vi "Disconnect.vi"(8 "error in (no error)":errorcluster, 11 "TCP Comm":T1) -> (0 "error out":errorcluster)   [LabVIEW 2020, in "TCP Comms.lvlib"]
uses:
  TCP Comms.lvlib
  TCP Comm.ctl
  Ref Data.ctl
  State.ctl
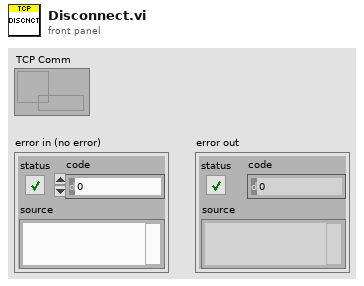
[diagram p1: front panel]
types:
  T1 = typedef "TCP Comms.lvlib/TCP Comm.ctl" = refnum<data-value>
  T2 = typedef "TCP Comms.lvlib/State.ctl" = enum16{"Idle", "Starting", "Connecting", "Connected", "Disconnecting", "Stopped"}
  T3 = typedef "TCP Comms.lvlib/Ref Data.ctl" = cluster{"TCP":refnum<k5>, "State":T2, "Server":bool, "Host":string, "Port":u16, "Listener":refnum<k5>, "Start":bool, "Disconnect":bool, "TCP Valid":bool, "TLS Enabled":bool, "Immutable TLS":refnum<k36>, "Certificate DN":string}
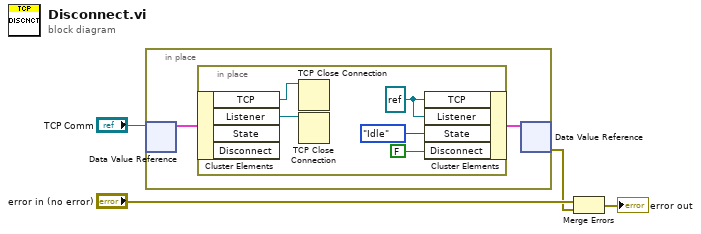
[diagram p0: block diagram]
diagram:
  n1 = in-place {
    n2 = in-place-dvr #1("TCP Comm") -> (w6:T3)  [unwired: 1 out]
    n3 = in-place {
      w9 = refnum<k5> refnum ("TCP")
      n4 = in-place-cluster #2(w6) -> ("TCP"=w10:refnum<k5>, "Listener"=w11:refnum<k5>)  [unwired: 2 out]
      n5 = TCP Close Connection(connection ID=w10) -> ()  [unwired: 2 in, 2 out]
      n6 = TCP Close Connection(connection ID=w11) -> ()  [unwired: 2 in, 2 out]
      n7 = in-place-cluster #2("TCP"=w9, "Listener"=w9, "State"=State."Idle", "Disconnect"=FALSE) -> (w5:T3)
    }
    n8 = in-place-dvr #1(w5) -> (w1:errorcluster)  [unwired: 1 out]
  }
  n9 = Merge Errors("error in (no error)", w1) -> (→"error out":errorcluster)
